vi "Desktop Main.vi"() -> ()   [LabVIEW 2021]
doc: "This example can view shared variable data that is published by RT Main.vi running on the myRIO device."
panel:
  in  "Tab Control":T1(tab)
  out "Accelerometer":waveform(dbl)[](graph)
  out "Audio":waveform(dbl)[](graph)
  out "LED3":bool
  out "LED2":bool
  out "LED1":bool
  out "LED0":bool
  out "DIO.A":waveform(u8)(graph)
  out "AI.A":waveform(dbl)[](graph)
  in  "DIO.A Input/Output":u16(ring) items=["Input", "Output"]
  in  "DIO Channel.A":u16(ring) items=["A/DIO0", "A/DIO1", "A/DIO2", "A/DIO3", "A/DIO4", "A/DIO5", "A/DIO6", "A/DIO7", "A/DIO8", "A/DIO9", "A/DIO10", "A/DIO11", "A/DIO12", "A/DIO13", "A/DIO14", "A/DIO15"]
  in  "AO Channel.A":enum16{"A/AO0", "A/AO1"}(ring)
  in  "AI Channel.A":enum16{"A/AI0", "A/AI1", "A/AI2", "A/AI3"}(ring)
  in  "DIO.B Input/Output":u16(ring) items=["Input", "Output"]
  in  "DIO Channel.B":u16(ring) items=["B/DIO0", "B/DIO1", "B/DIO2", "B/DIO3", "B/DIO4", "B/DIO5", "B/DIO6", "B/DIO7", "B/DIO8", "B/DIO9", "B/DIO10", "B/DIO11", "B/DIO12", "B/DIO13", "B/DIO14", "B/DIO15"]
  in  "AO Channel.B":u16(ring) items=["B/AO0", "B/AO1"]
  in  "AI Channel.B":enum16{"B/AI0", "B/AI1", "B/AI2", "B/AI3"}(ring)
  out "AI.B":waveform(dbl)[](graph)
  out "DIO.B":waveform(u8)(graph)
  out "AI.C":waveform(dbl)[](graph)
  in  "DIO.C Input/Output":u16(ring) items=["Input", "Output"]
  in  "DIO Channel.C":u16(ring) items=["C/DIO0", "C/DIO1", "C/DIO2", "C/DIO3", "C/DIO4", "C/DIO5", "C/DIO6", "C/DIO7"]
  in  "AO Channel.C":u16(ring) items=["C/AO0", "C/AO1"]
  in  "AI Channel.C":u16(ring) items=["C/AI0", "C/AI1"]
  out "DIO.C":waveform(u8)(graph)
  in  "stop":bool
  # "Overview: This example can view shared variable data that is published by RT Main.vi running on the myRIO device.\nRequirements: Network Variable Engine on the myRIO, Data Dashboard on iPad\nInstructions:\n1. Run RT Main.vi on the myRIO target.\n2. Run this VI."
  # "There are two ways to view the shared \nvariable data published by RT Main.vi that you \nrun on the myRIO:\n--View the data on iPad: You can find detailed \ninstructions in the readme file of the Data\nDashboard for myRIO example and the help file\nof Data Dashboard.\n--View the data on PC: Run RT Main.vi on the \nmyRIO, and run Desktop Main.vi. View the \nshared variable data in Desktop Main.vi."
  # "LED Status :"
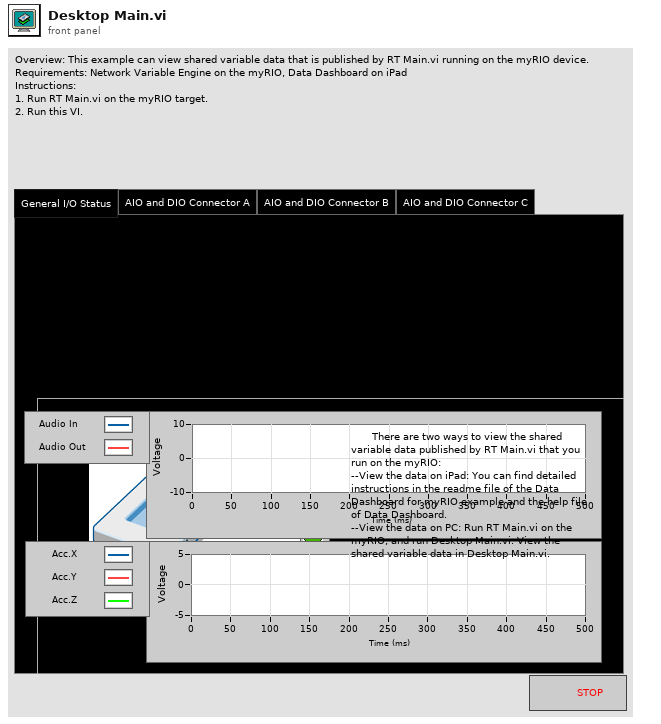
[diagram p1: front panel]
types:
  T1 = enum32{"General I/O Status", "AIO and DIO Connector A", "AIO and DIO Connector B", "AIO and DIO Connector C"}
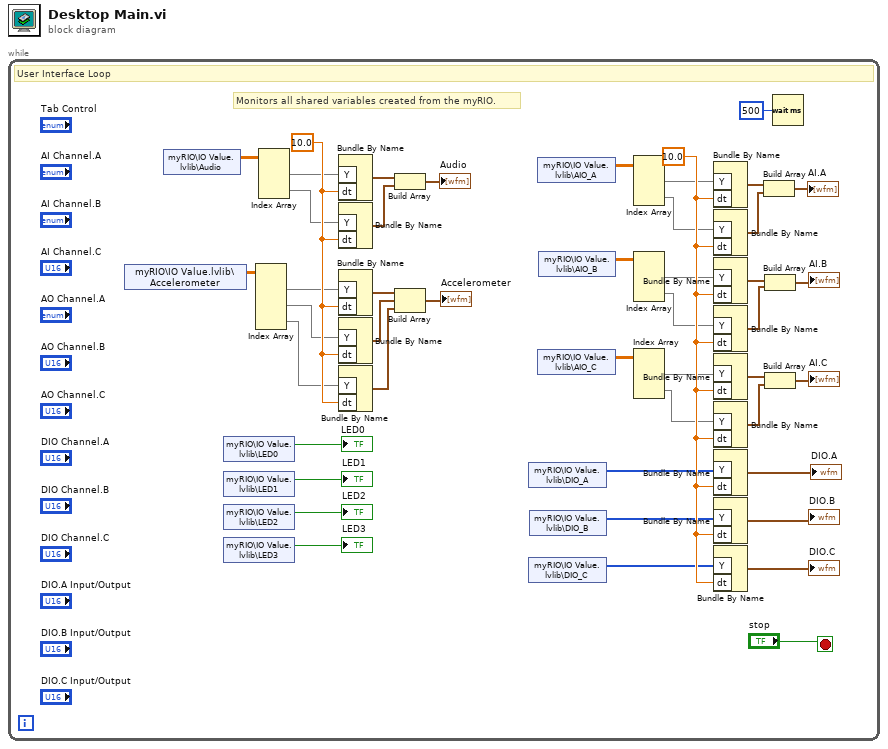
[diagram p0: block diagram]
diagram:
  n1 = while {
    stop <- "stop" stop-if-true
    w46 = 10.0 ("dt")
    w45 = 10.0 ("dt")
    # "Monitors all shared variables created from the myRIO."
    # "User Interface Loop"
    n2 = shared-variable "myRIO\\IO Value.lvlib\\Accelerometer"() -> (w30:dbl[][])  [unwired: 1 in, 1 out]
    n3 = shared-variable "myRIO\\IO Value.lvlib\\Audio"() -> (w33:dbl[][])  [unwired: 1 in, 1 out]
    n4 = shared-variable "myRIO\\IO Value.lvlib\\LED0"() -> (→"LED0":bool)  [unwired: 1 in, 1 out]
    n5 = shared-variable "myRIO\\IO Value.lvlib\\LED1"() -> (→"LED1":bool)  [unwired: 1 in, 1 out]
    n6 = shared-variable "myRIO\\IO Value.lvlib\\LED2"() -> (→"LED2":bool)  [unwired: 1 in, 1 out]
    n7 = shared-variable "myRIO\\IO Value.lvlib\\LED3"() -> (→"LED3":bool)  [unwired: 1 in, 1 out]
    n8 = Index Array(array=w30) -> (element #1=w29:dbl[], element #2=w28:dbl[], element #3=w27:dbl[])  [unwired: 6 in]
    n9 = Index Array(array=w33) -> (element #1=w32:dbl[], element #2=w31:dbl[])  [unwired: 4 in]
    n10 = Bundle By Name("Y"=w32, "dt"=w45) -> (w26:waveform(dbl))  [unwired: 1 in]
    n11 = Bundle By Name("Y"=w31, "dt"=w45) -> (w25:waveform(dbl))  [unwired: 1 in]
    n12 = Bundle By Name("Y"=w29, "dt"=w45) -> (w24:waveform(dbl))  [unwired: 1 in]
    n13 = Bundle By Name("Y"=w28, "dt"=w45) -> (w23:waveform(dbl))  [unwired: 1 in]
    n14 = Bundle By Name("Y"=w27, "dt"=w45) -> (w22:waveform(dbl))  [unwired: 1 in]
    n15 = Build Array(w26, w25) -> (→"Audio":waveform(dbl)[])
    n16 = Build Array(w24, w23, w22) -> (→"Accelerometer":waveform(dbl)[])
    n17 = shared-variable "myRIO\\IO Value.lvlib\\DIO_A"() -> (w36:u8[])  [unwired: 1 in, 1 out]
    n18 = shared-variable "myRIO\\IO Value.lvlib\\DIO_C"() -> (w34:u8[])  [unwired: 1 in, 1 out]
    n19 = shared-variable "myRIO\\IO Value.lvlib\\DIO_B"() -> (w35:u8[])  [unwired: 1 in, 1 out]
    n20 = shared-variable "myRIO\\IO Value.lvlib\\AIO_A"() -> (w21:dbl[][])  [unwired: 1 in, 1 out]
    n21 = shared-variable "myRIO\\IO Value.lvlib\\AIO_C"() -> (w15:dbl[][])  [unwired: 1 in, 1 out]
    n22 = shared-variable "myRIO\\IO Value.lvlib\\AIO_B"() -> (w18:dbl[][])  [unwired: 1 in, 1 out]
    n23 = Index Array(array=w21) -> (element #1=w20:dbl[], element #2=w19:dbl[])  [unwired: 4 in]
    n24 = Index Array(array=w18) -> (element #1=w17:dbl[], element #2=w16:dbl[])  [unwired: 4 in]
    n25 = Index Array(array=w15) -> (element #1=w14:dbl[], element #2=w13:dbl[])  [unwired: 4 in]
    n26 = Bundle By Name("Y"=w20, "dt"=w46) -> (w12:waveform(dbl))  [unwired: 1 in]
    n27 = Bundle By Name("Y"=w19, "dt"=w46) -> (w11:waveform(dbl))  [unwired: 1 in]
    n28 = Bundle By Name("Y"=w17, "dt"=w46) -> (w10:waveform(dbl))  [unwired: 1 in]
    n29 = Bundle By Name("Y"=w16, "dt"=w46) -> (w9:waveform(dbl))  [unwired: 1 in]
    n30 = Bundle By Name("Y"=w14, "dt"=w46) -> (w7:waveform(dbl))  [unwired: 1 in]
    n31 = Bundle By Name("Y"=w13, "dt"=w46) -> (w6:waveform(dbl))  [unwired: 1 in]
    n32 = Bundle By Name("Y"=w36, "dt"=w46) -> (→"DIO.A":waveform(u8))  [unwired: 1 in]
    n33 = Bundle By Name("Y"=w35, "dt"=w46) -> (→"DIO.B":waveform(u8))  [unwired: 1 in]
    n34 = Bundle By Name("Y"=w34, "dt"=w46) -> (→"DIO.C":waveform(u8))  [unwired: 1 in]
    n35 = Build Array(w12, w11) -> (→"AI.A":waveform(dbl)[])
    n36 = Build Array(w10, w9) -> (→"AI.B":waveform(dbl)[])
    n37 = Build Array(w7, w6) -> (→"AI.C":waveform(dbl)[])
    n38 = Wait (ms)(milliseconds to wait=u32 500) -> ()  [unwired: 1 out]
  }
